vi "Create.vi"(5 "Sequencer":refnum<class "MessageQ.lvclass">, 6 "State Control":T4, 7 "VolatusAPI":refnum<class "VolatusAPI.lvclass">, 8 "error in (no error)":refnum<class "MultiErrors.lvclass">, 10 "State":T1) -> (0 "error out":refnum<class "MultiErrors.lvclass">, 3 "State out":refnum<class "State.lvclass">)   [LabVIEW 2023, in "VolatusSeq.lvlib" / "State.lvclass"]
uses:
  State.lvclass
  VolatusErrorUtilities/MultiErrors/MultiErrors.lvclass
  State Control.ctl
  Sequence Time.ctl
  Variables/Variables.lvclass
  VolatusSeqConfig/State.ctl
  VolatusSeqConfig/Step.ctl
  VolatusSeqConfig/Command Config/Command Config.lvclass
  VolatusSeqConfig/Transition Config/Transition Config.lvclass
  VolatusSeqConfig/Debug Flags.ctl
  Volatus/VolatusAPI/VolatusAPI.lvclass
  Volatus/MessageQ/MessageQ.lvclass
  State.lvclass/State.ctl
  VolatusSeq.lvlib
  VolatusSeqConfig/VolatusSeqConfig.lvlib
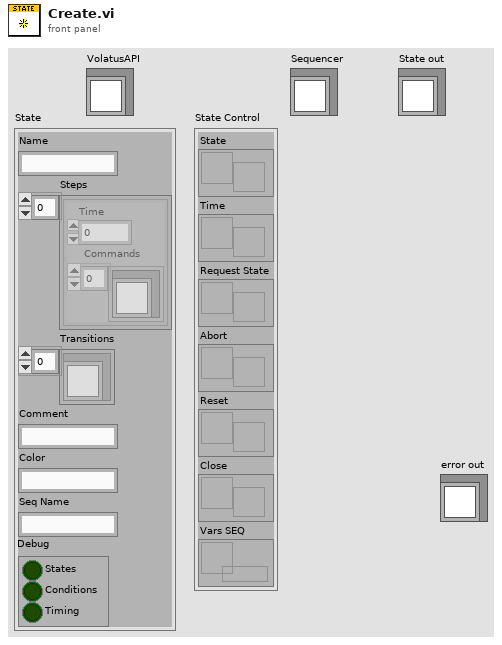
[diagram p1: front panel]
types:
  T1 = typedef "VolatusSeqConfig.lvlib/State.ctl" = cluster{"Name":string, "Steps":T2[], "Transitions":refnum<class "Transition Config.lvclass">[], "Comment":string, "Color":string, "Seq Name":string, "Debug":T3}
  T2 = typedef "VolatusSeqConfig.lvlib/Step.ctl" = cluster{"Time":dbl, "Commands":refnum<class "Command Config.lvclass">[]}
  T3 = typedef "VolatusSeqConfig.lvlib/Debug Flags.ctl" = cluster{"States":bool, "Conditions":bool, "Timing":bool}
  T4 = typedef "VolatusSeq.lvlib/State Control.ctl" = cluster{"State":refnum<notifier>, "Time":refnum<notifier>, "Request State":refnum<notifier>, "Abort":refnum<notifier>, "Reset":refnum<notifier>, "Close":refnum<notifier>, "Vars SEQ":refnum<queue>}
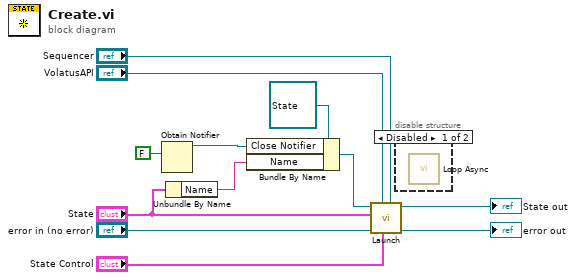
[diagram p0: block diagram]
diagram:
  n1 = Obtain Notifier(notification data type=FALSE) -> (notifier out=w5:refnum<notifier>)  [unwired: 3 in, 2 out]
  n2 = Unbundle By Name("State") -> ("Name"=w2:string)
  n3 = Bundle By Name(cluster=refnum<class "State.lvclass"> refnum ("State in"), "Close Notifier"=w5, "Name"=w2) -> (w6:refnum<class "State.lvclass">)
  n4 = call "Launch.vi"("Sequencer"="Sequencer", "State Control"="State Control", "VolatusAPI"="VolatusAPI", "error in (no error)"="error in (no error)", "State"="State", "State in"=w6) -> ("error out"=→"error out":refnum<class "MultiErrors.lvclass">, "State out"=→"State out":refnum<class "State.lvclass">)  [unwired: 4 in]
  n5 = disable-structure shown="Disabled" {
    frame Disabled {
      n6 = call "Loop Async.vi"() -> ()  [unwired: 12 in]
    }
    frame Enabled {
    }
  }
